vi "Perform Step.vi"(8 "error in (no error)":errorcluster, 11 "Timing Action in":refnum<class "Timing Action.lvclass">) -> (0 "error out":errorcluster, 2 "Result":T1, 3 "Timing Action out":refnum<class "Timing Action.lvclass">)   [LabVIEW 2020, in "MacroAssert.lvlib" / "Timing Action.lvclass"]
uses:
  Timing Action.lvclass
  CTLs/Report Data.ctl
  CTLs/FGV Actions.ctl
  <vilib>/Utility/error.llb/Error Cluster From Error Code.vi
  MacroAssert.lvlib
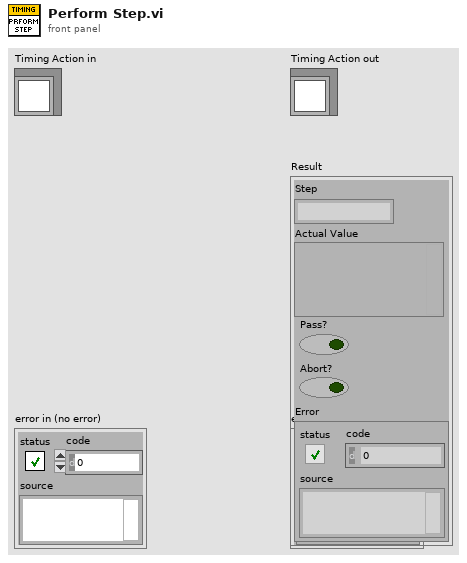
[diagram p1: front panel]
types:
  T1 = typedef "MacroAssert.lvlib/Report Data.ctl" = cluster{"Step":string, "Actual Value":variant, "Pass?":bool, "Abort?":bool, "Error":errorcluster}
  T2 = typedef "MacroAssert.lvlib/Timing Action.lvclass/Time Unit.ctl" = enum16{"milliseconds", "seconds", "minutes"}
  T3 = typedef "MacroAssert.lvlib/Timing Action.lvclass/Timing Action Type.ctl" = enum16{"Wait", "Wait Until"}
  T4 = typedef "MacroAssert.lvlib/FGV Actions.ctl" = enum16{"Read", "Write"}
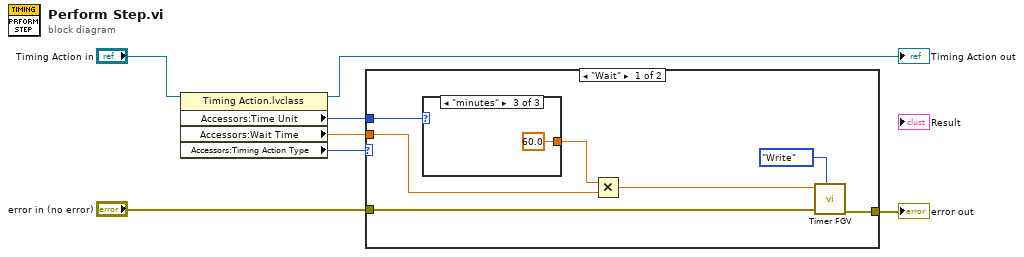
[diagram p0: block diagram]
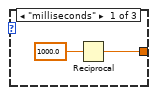
[diagram p2: hidden frame]
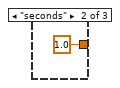
[diagram p3: hidden frame]
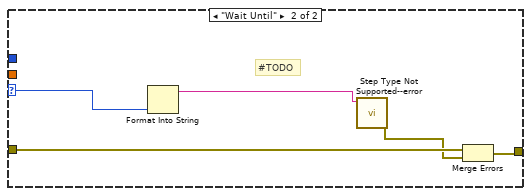
[diagram p4: hidden frame]
diagram:
  n1 = property class="Timing Action.lvclass"(reference="Timing Action in") -> (reference out=→"Timing Action out":refnum<class "Timing Action.lvclass">, "Accessors:Time Unit"=w1:T2, "Accessors:Wait Time"=w2:dbl, "Accessors:Timing Action Type"=w3:T3)  [unwired: 1 in, 1 out]
  n2 = case shown="\"Wait\"" w3 {
    selector: w3 -> [_ w20]
    tunnel: "error in (no error)" -> [w13 w23]
    tunnel: [w12 w21] -> w4
    tunnel: w2 -> [w9 _]
    tunnel: w1 -> [w11 _]
    frame "Wait" {
      n3 = case shown="\"minutes\"" w11 {
        tunnel: [w15 1.0 60.0] -> w10
        frame "milliseconds" {
          n4 = Reciprocal(x=1000.0) -> (1/x=w15:dbl)
        }
        frame "seconds" {
        }
        frame "minutes" {
        }
      }
      n5 = Multiply(x=w10, y=w9) -> (x*y=w8:dbl)
      n6 = call "Timer FGV.vi"("Mode"=FGV_Actions."Write", "error in (no error)"=w13, "Timer Value (s)"=w8) -> ("error out"=w12:errorcluster)  [unwired: 6 in, 2 out]
    }
    frame "Wait Until" {
      # "#TODO"
      n7 = Format Into String(w20) -> (resulting string=w19:string)  [unwired: 3 in, 1 out]
      n8 = call "Step Type Not Supported--error.vi"("Step Type"=w19) -> ("error out"=w22:errorcluster)  [unwired: 10 in]
      n9 = Merge Errors(w23, w22) -> (w21:errorcluster)
    }
  }
  "error out" <- w4
